vi "Copy Template Source to New Location.vi"(8 "error in":errorcluster, 10 "destination directory (default data directory if empty)":path, 11 "custom device name":string) -> (0 "error out":errorcluster, 3 "custom device path out":path)   [LabVIEW 2020, in "Template Tool.lvlib"]
uses:
  Template Tool.lvlib
  Template Tool Global.vi
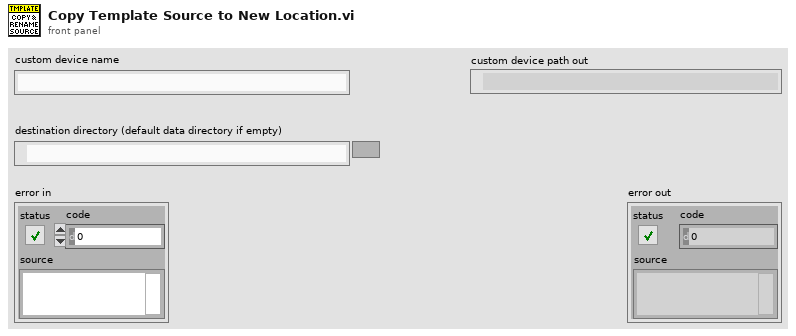
[diagram p1: front panel]
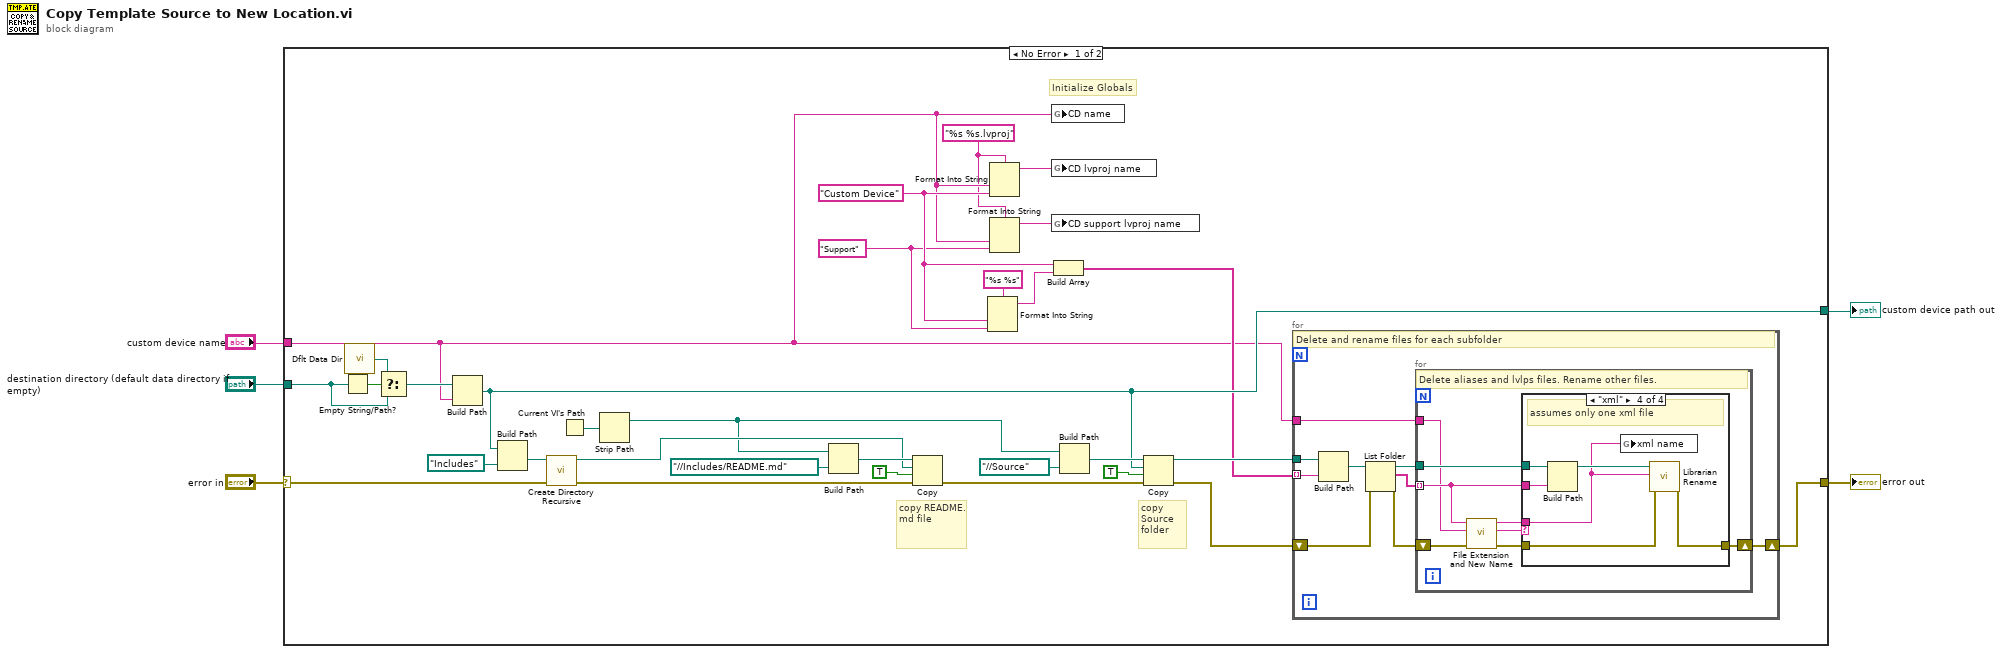
[diagram p0: block diagram]
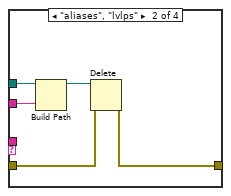
[diagram p3: hidden frame]
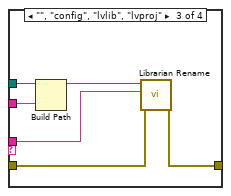
[diagram p4: hidden frame]
diagram:
  n1 = case shown="No Error" "error in" {
    selector: "error in" -> [w18 w72]
    tunnel: "destination directory (default data directory if empty)" -> [w34 _]
    tunnel: [w32 w72] -> w4
    tunnel: [w23 _] -> w3
    tunnel: "custom device name" -> [w8 _]
    frame No Error {
      w6 = "%s %s.lvproj" ("name or relative path")
      w11 = "Custom Device" ("name or relative path")
      w10 = "Support" ("name or relative path")
      # "Initialize Globals"
      # "copy Source folder"
      # "copy README.md file"
      n2 = Empty String/Path?(string/path=w34) -> (empty?=w36:bool)
      n3 = call <vilib>:"Dflt Data Dir.vi"() -> ("App:Default Data Directory"=w35:path)
      n4 = Select(t=w35, s=w36, f=w34) -> (s? t:f=w17:path)
      n5 = Build Path(base path=w17, name or relative path=w8) -> (appended path=w23:path)
      n6 = Build Path(base path=w23, name or relative path=path "Includes") -> (appended path=w22:path)
      n7 = call <vilib>:"Create Directory Recursive.vi"("error in (no error)"=w18, "directory"=w22) -> ("error out"=w25:errorcluster, "directory copy"=w21:path)  [unwired: 3 in, 1 out]
      n8 = Current VI's Path() -> (path=w20:path)
      n9 = Strip Path(path=w20) -> (stripped path=w19:path)  [unwired: 1 out]
      n10 = Build Path(base path=w19, name or relative path=path "../../Includes/README.md") -> (appended path=w30:path)
      n11 = Copy(8:w25, 9:TRUE ("overwrite (F)"), 10:w21, 11:w30) -> (0:w26:errorcluster)  [unwired: 1 in, 2 out]
      n12 = Format Into String(format string="%s %s", w11, w10) -> (resulting string=w12:string)  [unwired: 2 in, 1 out]
      n13 = Format Into String(format string=w6, w8, w11) -> (resulting string=w9:string)  [unwired: 2 in, 1 out]
      n14 = Format Into String(format string=w6, w8, w10) -> (resulting string=w7:string)  [unwired: 2 in, 1 out]
      n15 = global write "Template Tool Global.vi" "CD name"(w8) -> ()
      n16 = global write "Template Tool Global.vi" "CD lvproj name"(w9) -> ()
      n17 = global write "Template Tool Global.vi" "CD support lvproj name"(w7) -> ()
      n18 = Build Array(w11, w12) -> (w14:string[])
      n19 = Build Path(base path=w19, name or relative path=path "../../Source") -> (appended path=w29:path)
      n20 = Copy(8:w26, 9:TRUE ("overwrite (F)"), 10:w23, 11:w29) -> (0:w16:errorcluster, 3:w15:path)  [unwired: 1 in, 1 out]
      n21 = for {
        tunnel: w8 -> [w43]
        tunnel: w15 -> [w40]
        shift-right: [w42] -> w32
        shift-left: w16 -> [w37]
        tunnel: w14 -> [w38] mode=indexing
        # "Delete and rename files for each subfolder"
        n22 = Build Path(base path=w40, name or relative path=w38) -> (appended path=w41:path)
        n23 = List Folder(path=w41, error in=w37) -> (path out=w39:path, filenames=w45:string[], error out=w44:errorcluster)  [unwired: 2 in, 1 out]
        n24 = for {
          tunnel: w39 -> [w53]
          tunnel: w45 -> [w51] mode=indexing
          shift-right: [w52] -> w42
          shift-left: w44 -> [w47]
          tunnel: w43 -> [w48]
          # "Delete aliases and lvlps files. Rename other files."
          n25 = call "File Extension and New Name.vi"("error in"=w47, "custom device name"=w48, "filename"=w51) -> ("error out"=w46:errorcluster, "extension"=w49:string, "new filename"=w50:string)  [unwired: 6 in]
          n26 = case shown="\"xml\"" w49 {
            tunnel: w53 -> [_ w58 w65 w71]
            tunnel: w51 -> [_ w57 w64 w70]
            tunnel: w46 -> [w54 w56 w63 w69]
            tunnel: [w54 w55 w62 w68] -> w52
            tunnel: w50 -> [_ _ w60 w66]
            frame Default {
            }
            frame "aliases", "lvlps" {
              n27 = Build Path(base path=w58, name or relative path=w57) -> (appended path=w59:path)
              n28 = Delete(path (use dialog)=w59, error in=w56) -> (error out=w55:errorcluster)  [unwired: 3 in, 2 out]
            }
            frame "", "config", "lvlib", "lvproj" {
              n29 = Build Path(base path=w65, name or relative path=w64) -> (appended path=w61:path)
              n30 = call <vilib>:"Librarian Rename.vi"("error in (no error)"=w63, "new name"=w60, "path"=w61) -> ("error out"=w62:errorcluster)  [unwired: 7 in, 1 out]
            }
            frame "xml" {
              # "assumes only one xml file"
              n31 = Build Path(base path=w71, name or relative path=w70) -> (appended path=w67:path)
              n32 = global write "Template Tool Global.vi" "xml name"(w66) -> ()
              n33 = call <vilib>:"Librarian Rename.vi"("error in (no error)"=w69, "new name"=w66, "path"=w67) -> ("error out"=w68:errorcluster)  [unwired: 7 in, 1 out]
            }
          }
        }
      }
    }
    frame Error {
    }
  }
  "custom device path out" <- w3
  "error out" <- w4
